vi "Do.vi"(8 "error in (no error)":errorcluster, 10 "Actor in":refnum<class "Actor.lvclass">, 11 "fire error object Msg":refnum<class "fire error object Msg.lvclass">) -> (0 "error out":errorcluster, 2 "Actor out":refnum<class "Actor.lvclass">)   [LabVIEW 2020, in "Template.lvlib" / "fire error object Msg.lvclass"]
doc: "This VI delivers the message to the actor by calling the appropriate method(s) on the actor."
uses:
  fire error object Msg.lvclass
  <vilib>/ActorFramework/Actor/Actor.lvclass
  fire error object Msg.lvclass/fire error object Msg.ctl
  template/Template.lvclass
  C:/Program Files/National Instruments/LabVIEW 2020/vi.lib/ActorFramework/Actor/Actor.lvclass
  template/Template.lvclass/Template.ctl
  9ef47adc-f318-494c-9b8b-6df3216d6863.vi
  template/accessors/Read Actor Events.vi
  <vilib>/Utility/error.llb/Clear Errors.vi
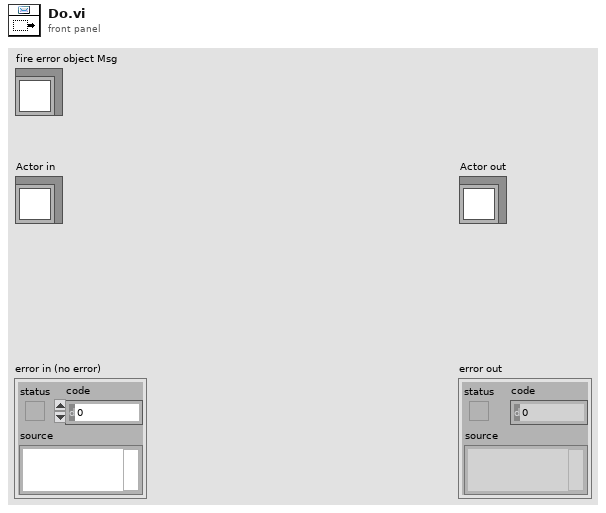
[diagram p1: front panel]
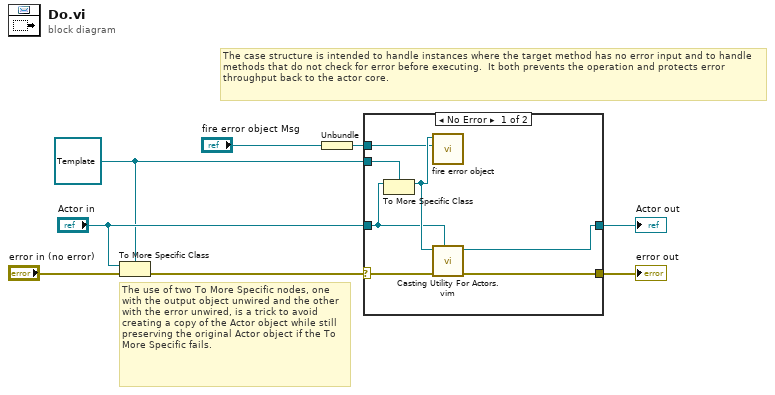
[diagram p0: block diagram]
diagram:
  w2 = refnum<class "Template.lvclass"> refnum ("Actor in")
  # "The use of two To More Specific nodes, one with the output object unwired and the other with the error unwired, is a trick to avoid creating a copy of the Actor object while still preserving the original Actor object if the To More Specific fails."
  # "The case structure is intended to handle instances where the target method has no error input and to handle methods that do not check for error before executing.  It both prevents the operation and protects error throughput back to the actor core."
  n1 = To More Specific Class(target class=w2, reference="Actor in", error in="error in (no error)") -> (error out=w6:errorcluster)  [unwired: 1 out]
  n2 = Unbundle("fire error object Msg") -> (w1:refnum<class>)
  n3 = case shown="No Error" w6 {
    selector: w6 -> [w15 w17]
    tunnel: [w10 w17] -> w5
    tunnel: [w11 w16] -> w4
    tunnel: "Actor in" -> [w12 w16]
    tunnel: w2 -> [w13 _]
    tunnel: w1 -> [w9 _]
    frame No Error {
      n4 = To More Specific Class(target class=w13, reference=w12) -> (specific class reference=w14:refnum<class "Template.lvclass">)  [unwired: 1 in, 1 out]
      n5 = call "fire error object.vi"("Error in"=w9, "Template in"=w14) -> ()  [unwired: 10 in]
      n6 = call "Casting Utility For Actors.vim"("type"=w12, "error in (no error)"=w15, "Actor in"=w14) -> ("error out"=w10:errorcluster, "Actor out"=w11:refnum<class "Actor.lvclass">)  [unwired: 7 in]
    }
    frame Error {
      # "If type check fails, pass the original object out again."
    }
  }
  "error out" <- w5
  "Actor out" <- w4
